vi "Modbus_RTU_Setting.vi"(0 "VISA resource name":refnum<visa-resource-name>="COM18", 1 "Serial Config":T1={"baud rate (bps)"=9600, "stop bits"=10, "parity"=0, "flow control"=0, "timeout"=1000, "retries"=1} {"stop bits" items=["1.0"=10, "1.5"=15, "2.0"=20]; "parity" items=["None", "Odd", "Even", "Mark", "Space"]; "flow control" items=["None", "XON/XOFF", "RTS/CTS", "XON/XOFF & RTS/CTS", "DTR/DSR", "XON/XOFF & DTR/DSR"]}, 2 "address":u16=1, 4 "Registers In":u16[](array[numeric])=[1, 0, 2, 0, 0, 0, 0, 0, 0, 9], 5 "error in (no error)":errorcluster, 6 "Function":T2=enum."Read Holding Register03", 7 "Coil Single value":bool=TRUE, 8 "quantity":u16=2, 9 "Register Single Value":u16=100) -> (19 "error out":errorcluster={"status"=FALSE, "code"=-1073807339, "source"="VISA Read in MB Master.lvlib:MB_ADU_RTU.lvclass:RX ADU.vi:4960001->MB Master.lvlib:MB_Master_Serial.lvclass:Querry.vi:3550001->MB Master.lvlib:Read Holding Registers.vi:2420001->Modbus_RTU_Setting.vi"})   [LabVIEW 2024]
uses:
  Modbus Control.ctl
  <vilib>/Plasmionique/MB Master/MB_Master_Serial/MB_Master_Serial.lvclass
  C:/Program Files (x86)/National Instruments/LabVIEW 2024/vi.lib/Plasmionique/MB Master/MB_Master/MB_Master.lvclass
  <vilib>/Plasmionique/MB Master/MB Master.lvlib
panel:
  out "(hi.lo)":dbl
  out "Registers":u16[](array[numeric])
  out "Coils Outputs":bool[](array[boolean])
  in  "Coils In":bool[](array[boolean])=[TRUE, TRUE, FALSE, FALSE, FALSE, FALSE, FALSE, FALSE, TRUE, TRUE]
  # "Modbus RTU Setting"
  # "Ver1.00"
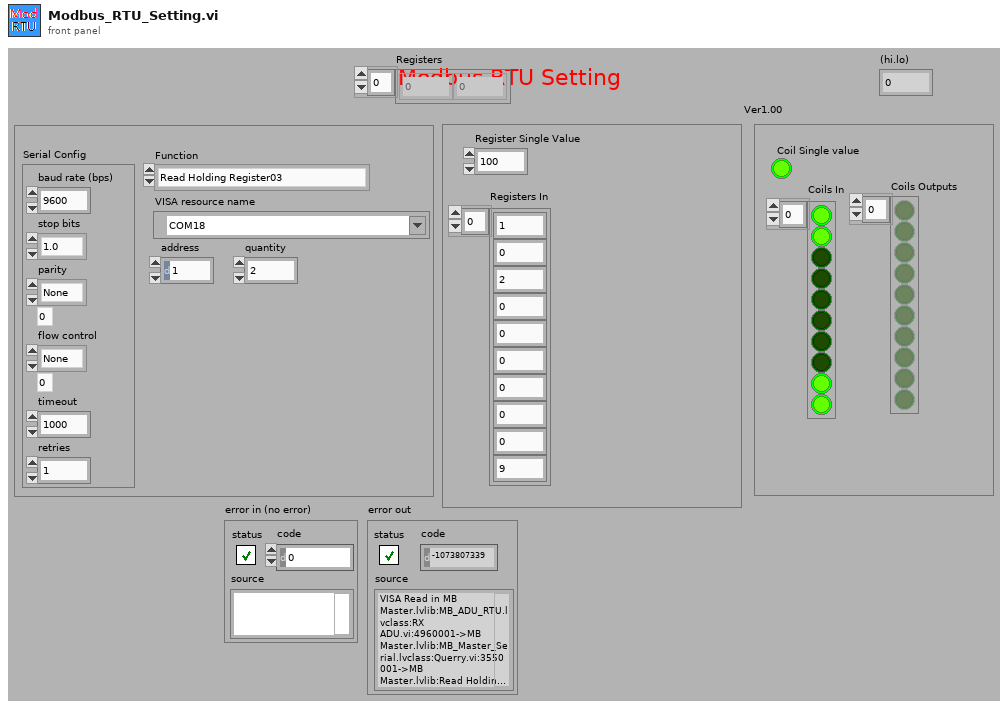
[diagram p1: front panel]
types:
  T1 = cluster{"baud rate (bps)":u32, "stop bits":u16, "parity":u16, "flow control":u16, "timeout":u32, "retries":i32}
  T2 = typedef "Modbus Control.ctl" = enum16{"Read Coils01", "Read Discrete Input02", "Read Holding Register03", "Read Input Registers04", "Write Single Coil05", "Write Single Register06", "Write Multiple Coils15", "Write Multiple Registers16"}
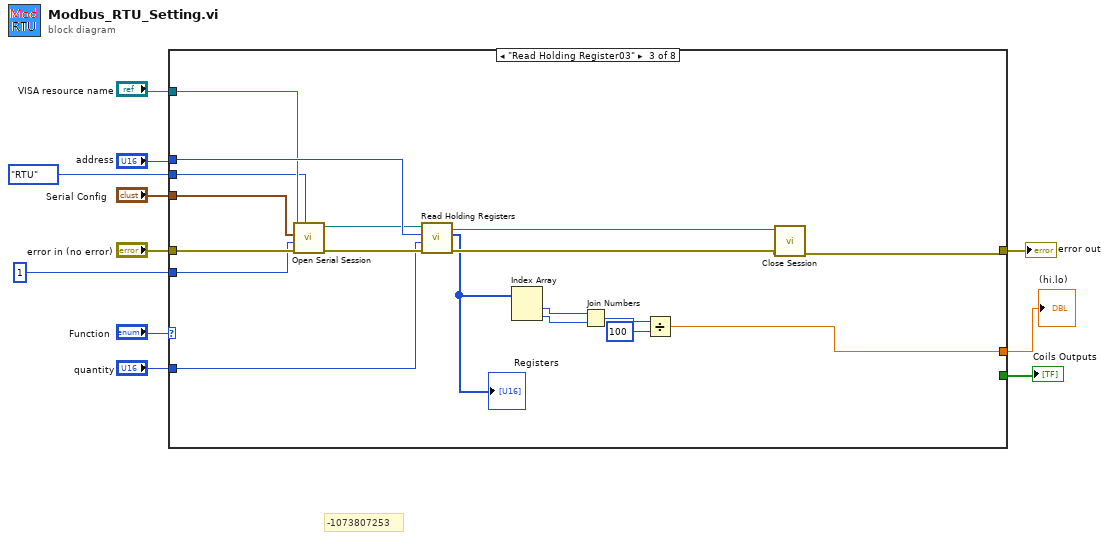
[diagram p0: block diagram]
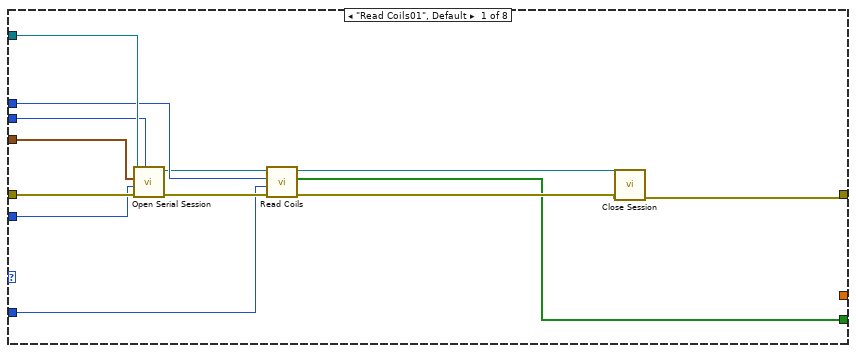
[diagram p2: hidden frame]
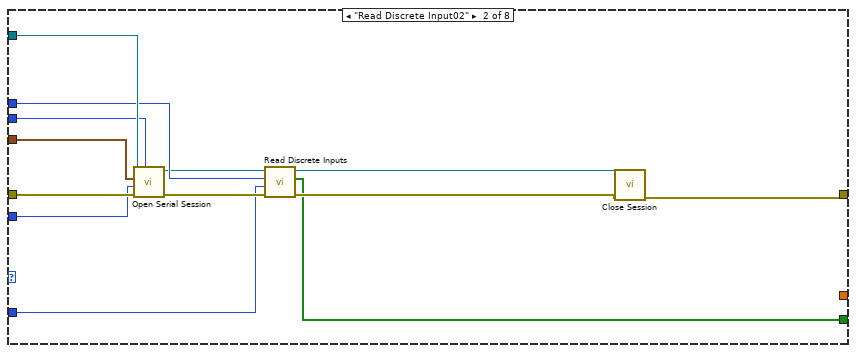
[diagram p3: hidden frame]
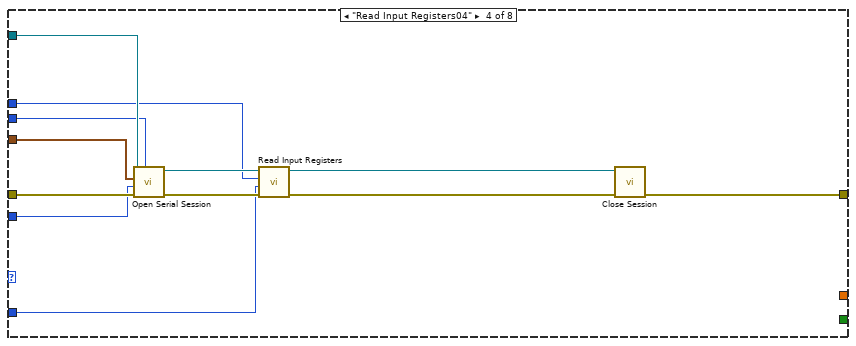
[diagram p4: hidden frame]
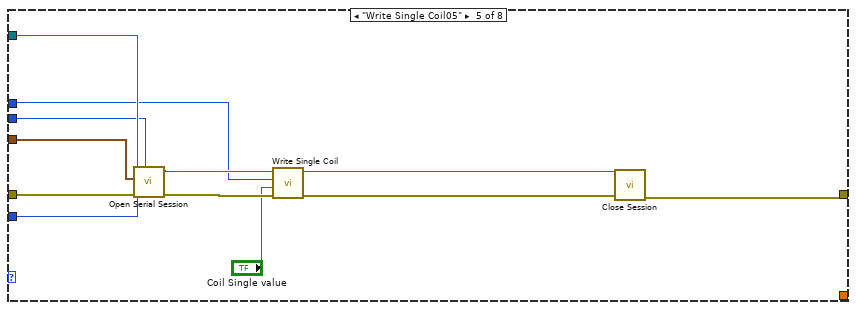
[diagram p5: hidden frame]
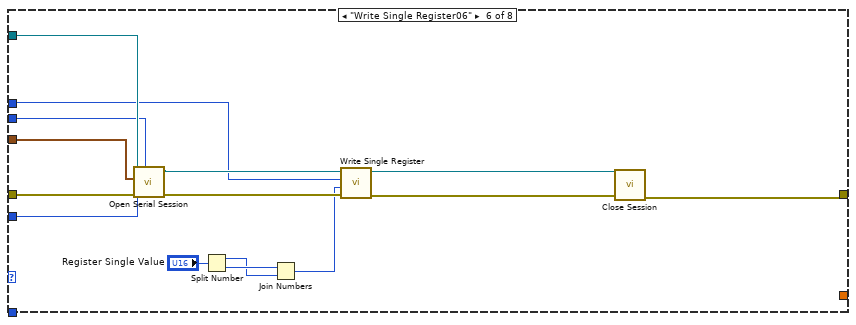
[diagram p6: hidden frame]
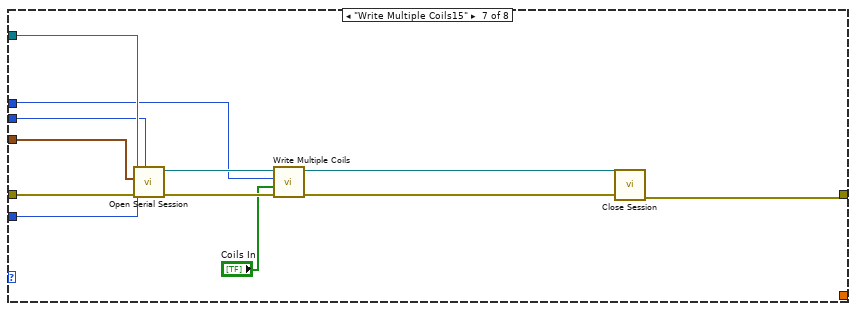
[diagram p7: hidden frame]
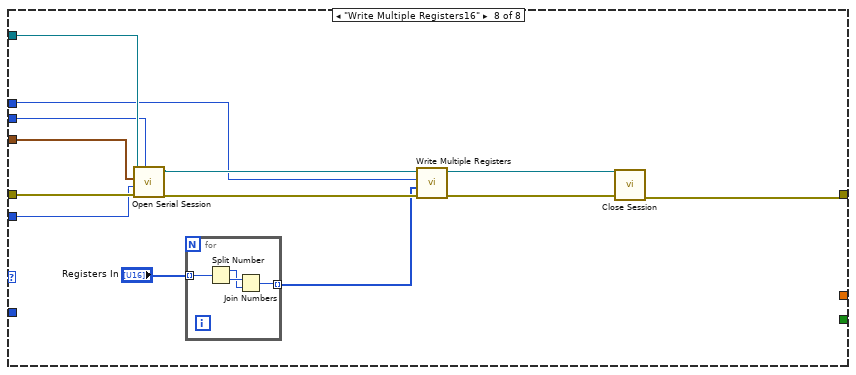
[diagram p8: hidden frame]
diagram:
  # "-1073807253"
  n1 = case shown="\"Read Holding Register03\"" "Function" {
    tunnel: "VISA resource name" -> [w23 w36 w53 w66 w78 w93 w105 w118]
    tunnel: "Serial Config" -> [w22 w35 w52 w65 w77 w92 w104 w117]
    tunnel: "error in (no error)" -> [w24 w37 w54 w67 w79 w94 w106 w119]
    tunnel: [w21 w34 w47 w64 w76 w91 w103 w116] -> w8
    tunnel: "address" -> [w15 w28 w55 w57 w69 w87 w96 w111]
    tunnel: enum16{"RTU", "ASCII"}."RTU" ("Mode (RTU)") -> [w20 w33 w46 w63 w75 w85 w102 w110]
    tunnel: u8 1 ("Slave ID") -> [w19 w32 w45 w62 w74 w84 w101 w109]
    tunnel: "quantity" -> [w16 w29 w44 w56 _ _ _ _]
    tunnel: [w12 w25 _ _ _ _ _ _] -> w2
    tunnel: [_ _ w38 _ _ _ _ _] -> w1
    frame "Read Coils01", Default {
      n2 = call <vilib>:"Open Serial Session.vi"("Mode (RTU)"=w20, "Error in"=w24, "Slave ID"=w19, "Serial Config"=w22, "VISA Resource"=w23) -> ("Error out"=w17:errorcluster, "MB_Serial session"=w14:refnum<class "MB_Master_Serial.lvclass">)  [unwired: 5 in]
      n3 = call <vilib>:"Read Coils.vi"("error in (no error)"=w17, "quantity"=w16, "starting address"=w15, "MB session in"=w14) -> ("error out"=w18:errorcluster, "Coils"=w12:bool[], "MB session out"=w13:refnum<class "MB_Master_Serial.lvclass">)  [unwired: 5 in]
      n4 = call-dynamic "Close Session.vi"("error in (no error)"=w18, "MB_Serial session"=w13) -> ("error out"=w21:errorcluster)  [unwired: 9 in]
    }
    frame "Read Discrete Input02" {
      n5 = call <vilib>:"Open Serial Session.vi"("Mode (RTU)"=w33, "Error in"=w37, "Slave ID"=w32, "Serial Config"=w35, "VISA Resource"=w36) -> ("Error out"=w30:errorcluster, "MB_Serial session"=w27:refnum<class "MB_Master_Serial.lvclass">)  [unwired: 5 in]
      n6 = call <vilib>:"Read Discrete Inputs.vi"("error in (no error)"=w30, "quantity"=w29, "starting address"=w28, "MB session in"=w27) -> ("error out"=w31:errorcluster, "Inputs"=w25:bool[], "MB session out"=w26:refnum<class "MB_Master_Serial.lvclass">)  [unwired: 5 in]
      n7 = call-dynamic "Close Session.vi"("error in (no error)"=w31, "MB_Serial session"=w26) -> ("error out"=w34:errorcluster)  [unwired: 9 in]
    }
    frame "Read Holding Register03" {
      n8 = call <vilib>:"Open Serial Session.vi"("Mode (RTU)"=w46, "Error in"=w54, "Slave ID"=w45, "Serial Config"=w52, "VISA Resource"=w53) -> ("Error out"=w51:errorcluster, "MB_Serial session"=w50:refnum<class "MB_Master_Serial.lvclass">)  [unwired: 5 in]
      n9 = call <vilib>:"Read Holding Registers.vi"("error in (no error)"=w51, "quantity"=w44, "starting address"=w55, "MB session in"=w50) -> ("error out"=w49:errorcluster, "Registers"=w43:u16[], "MB session out"=w48:refnum<class "MB_Master_Serial.lvclass">)  [unwired: 5 in]
      "Registers" <- w43
      n10 = Index Array(array=w43) -> (element #1=w42:u16, element #2=w41:u16)  [unwired: 2 in]
      n11 = Join Numbers(hi=w42, lo=w41) -> ((hi.lo)=w40:u32)
      n12 = Divide(x=w40, y=u32 100) -> (x/y=w38:dbl)
      n13 = call-dynamic "Close Session.vi"("error in (no error)"=w49, "MB_Serial session"=w48) -> ("error out"=w47:errorcluster)  [unwired: 9 in]
    }
    frame "Read Input Registers04" {
      n14 = call <vilib>:"Open Serial Session.vi"("Mode (RTU)"=w63, "Error in"=w67, "Slave ID"=w62, "Serial Config"=w65, "VISA Resource"=w66) -> ("Error out"=w60:errorcluster, "MB_Serial session"=w59:refnum<class "MB_Master_Serial.lvclass">)  [unwired: 5 in]
      n15 = call <vilib>:"Read Input Registers.vi"("error in (no error)"=w60, "quantity"=w56, "starting address"=w57, "MB session in"=w59) -> ("error out"=w61:errorcluster, "MB session out"=w58:refnum<class "MB_Master_Serial.lvclass">)  [unwired: 5 in, 1 out]
      n16 = call-dynamic "Close Session.vi"("error in (no error)"=w61, "MB_Serial session"=w58) -> ("error out"=w64:errorcluster)  [unwired: 9 in]
    }
    frame "Write Single Coil05" {
      n17 = call <vilib>:"Open Serial Session.vi"("Mode (RTU)"=w75, "Error in"=w79, "Slave ID"=w74, "Serial Config"=w77, "VISA Resource"=w78) -> ("Error out"=w72:errorcluster, "MB_Serial session"=w71:refnum<class "MB_Master_Serial.lvclass">)  [unwired: 5 in]
      n18 = call <vilib>:"Write Single Coil.vi"("error in (no error)"=w72, "value"="Coil Single value", "address"=w69, "MB session in"=w71) -> ("error out"=w73:errorcluster, "MB session out"=w70:refnum<class "MB_Master_Serial.lvclass">)  [unwired: 6 in]
      n19 = call-dynamic "Close Session.vi"("error in (no error)"=w73, "MB_Serial session"=w70) -> ("error out"=w76:errorcluster)  [unwired: 9 in]
    }
    frame "Write Single Register06" {
      n20 = call <vilib>:"Open Serial Session.vi"("Mode (RTU)"=w85, "Error in"=w94, "Slave ID"=w84, "Serial Config"=w92, "VISA Resource"=w93) -> ("Error out"=w86:errorcluster, "MB_Serial session"=w88:refnum<class "MB_Master_Serial.lvclass">)  [unwired: 5 in]
      n21 = Split Number(x="Register Single Value") -> (hi(x)=w81:u8, lo(x)=w83:u8)
      n22 = Join Numbers(hi=w83, lo=w81) -> ((hi.lo)=w80:u16)
      n23 = call <vilib>:"Write Single Register.vi"("error in (no error)"=w86, "value"=w80, "address"=w87, "MB session in"=w88) -> ("error out"=w90:errorcluster, "MB session out"=w89:refnum<class "MB_Master_Serial.lvclass">)  [unwired: 6 in]
      n24 = call-dynamic "Close Session.vi"("error in (no error)"=w90, "MB_Serial session"=w89) -> ("error out"=w91:errorcluster)  [unwired: 9 in]
    }
    frame "Write Multiple Coils15" {
      n25 = call <vilib>:"Open Serial Session.vi"("Mode (RTU)"=w102, "Error in"=w106, "Slave ID"=w101, "Serial Config"=w104, "VISA Resource"=w105) -> ("Error out"=w99:errorcluster, "MB_Serial session"=w98:refnum<class "MB_Master_Serial.lvclass">)  [unwired: 5 in]
      n26 = call <vilib>:"Write Multiple Coils.vi"("error in (no error)"=w99, "values"="Coils In", "starting address"=w96, "MB session in"=w98) -> ("error out"=w100:errorcluster, "MB session out"=w97:refnum<class "MB_Master_Serial.lvclass">)  [unwired: 6 in]
      n27 = call-dynamic "Close Session.vi"("error in (no error)"=w100, "MB_Serial session"=w97) -> ("error out"=w103:errorcluster)  [unwired: 9 in]
    }
    frame "Write Multiple Registers16" {
      n28 = call <vilib>:"Open Serial Session.vi"("Mode (RTU)"=w110, "Error in"=w119, "Slave ID"=w109, "Serial Config"=w117, "VISA Resource"=w118) -> ("Error out"=w114:errorcluster, "MB_Serial session"=w113:refnum<class "MB_Master_Serial.lvclass">)  [unwired: 5 in]
      n29 = for {
        tunnel: "Registers In" -> [w121] mode=indexing
        tunnel: [w120] -> w107 mode=indexing
        n30 = Split Number(x=w121) -> (hi(x)=w122:u8, lo(x)=w123:u8)
        n31 = Join Numbers(hi=w123, lo=w122) -> ((hi.lo)=w120:u16)
      }
      n32 = call <vilib>:"Write Multiple Registers.vi"("error in (no error)"=w114, "values"=w107, "starting address"=w111, "MB session in"=w113) -> ("error out"=w115:errorcluster, "MB session out"=w112:refnum<class "MB_Master_Serial.lvclass">)  [unwired: 6 in]
      n33 = call-dynamic "Close Session.vi"("error in (no error)"=w115, "MB_Serial session"=w112) -> ("error out"=w116:errorcluster)  [unwired: 9 in]
    }
  }
  "error out" <- w8
  "Coils Outputs" <- w2
  "(hi.lo)" <- w1
